vi "KH7008 Set All.vi"(8 "error in (no error)":errorcluster, 10 "Set All":T1={"Channel"=enum."Channel 2", "Gain"=enum."10x", "Bandwidth Filter"=enum."ON", "Shunt Resistor"=enum."50 Ohms", "Coupling"=enum."DC", "Input Config"=enum."Differential"}, 11 "VISA Refnum in":refnum<visa-resource-name>="COM1") -> (0 "error out":errorcluster)   [LabVIEW 2016, in "KH7008.lvclass"]
uses:
  KH7008.lvclass
  typedefs/SetAll-Cluster.ctl
  typedefs/Channel-Enum.ctl
  typedefs/Gain-Enum.ctl
  typedefs/Filter-Enum.ctl
  typedefs/Shunt-Enum.ctl
  typedefs/Coupling-Enum.ctl
  typedefs/Input Configuration-Enum.ctl
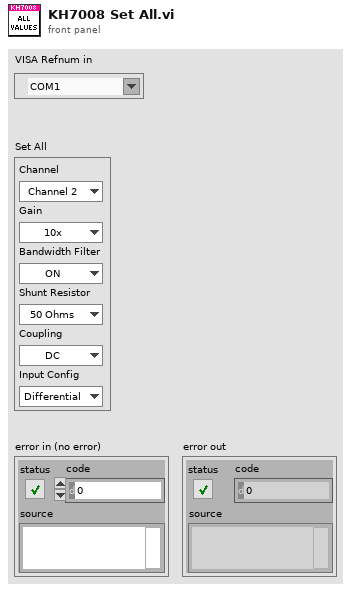
[diagram p1: front panel]
types:
  T1 = typedef "KH7008.lvclass/SetAll-Cluster.ctl" = cluster{"Channel":T2, "Gain":T3, "Bandwidth Filter":T4, "Shunt Resistor":T5, "Coupling":T6, "Input Config":T7}
  T2 = typedef "KH7008.lvclass/Channel-Enum.ctl" = enum16{"Channel 1", "Channel 2", "Channel 3", "Channel 4", "Channel 5", "Channel 6", "Channel 7", "Channel 8"}
  T3 = typedef "KH7008.lvclass/Gain-Enum.ctl" = enum16{"1x", "10x", "100x", "1000x"}
  T4 = typedef "KH7008.lvclass/Filter-Enum.ctl" = enum16{"OFF", "ON"}
  T5 = typedef "KH7008.lvclass/Shunt-Enum.ctl" = enum16{"Open", "50 Ohms", "500 Ohms", "5k Ohms", "50k Ohms"}
  T6 = typedef "KH7008.lvclass/Coupling-Enum.ctl" = enum16{"AC", "DC"}
  T7 = typedef "KH7008.lvclass/Input Configuration-Enum.ctl" = enum16{"Ground", "SE+ (-gnd)", "SE- (+gnd)", "Differential"}
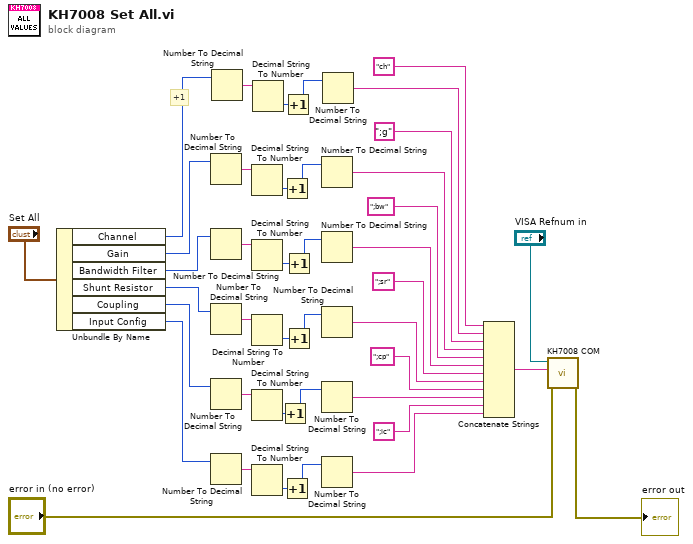
[diagram p0: block diagram]
diagram:
  # "+1"
  n1 = Unbundle By Name("Set All") -> ("Channel"=w6:T2, "Gain"=w33:T3, "Bandwidth Filter"=w32:T4, "Shunt Resistor"=w30:T5, "Coupling"=w31:T6, "Input Config"=w34:T7)
  n2 = Number To Decimal String(number=w33) -> (decimal integer string=w29:string)  [unwired: 1 in]
  n3 = Number To Decimal String(number=w32) -> (decimal integer string=w28:string)  [unwired: 1 in]
  n4 = Number To Decimal String(number=w30) -> (decimal integer string=w27:string)  [unwired: 1 in]
  n5 = Number To Decimal String(number=w31) -> (decimal integer string=w26:string)  [unwired: 1 in]
  n6 = Number To Decimal String(number=w34) -> (decimal integer string=w25:string)  [unwired: 1 in]
  n7 = Number To Decimal String(number=w6) -> (decimal integer string=w7:string)  [unwired: 1 in]
  n8 = Decimal String To Number(string=w29) -> (number=w24:i32)  [unwired: 2 in, 1 out]
  n9 = Decimal String To Number(string=w28) -> (number=w23:i32)  [unwired: 2 in, 1 out]
  n10 = Decimal String To Number(string=w27) -> (number=w20:i32)  [unwired: 2 in, 1 out]
  n11 = Decimal String To Number(string=w26) -> (number=w21:i32)  [unwired: 2 in, 1 out]
  n12 = Decimal String To Number(string=w25) -> (number=w22:i32)  [unwired: 2 in, 1 out]
  n13 = Decimal String To Number(string=w7) -> (number=w8:i32)  [unwired: 2 in, 1 out]
  n14 = Increment(x=w21) -> (x+1=w18:i32)
  n15 = Increment(x=w24) -> (x+1=w15:i32)
  n16 = Increment(x=w22) -> (x+1=w19:i32)
  n17 = Increment(x=w8) -> (x+1=w9:i32)
  n18 = Increment(x=w23) -> (x+1=w16:i32)
  n19 = Increment(x=w20) -> (x+1=w17:i32)
  n20 = Number To Decimal String(number=w15) -> (decimal integer string=w14:string)  [unwired: 1 in]
  n21 = Number To Decimal String(number=w16) -> (decimal integer string=w13:string)  [unwired: 1 in]
  n22 = Number To Decimal String(number=w17) -> (decimal integer string=w12:string)  [unwired: 1 in]
  n23 = Number To Decimal String(number=w18) -> (decimal integer string=w11:string)  [unwired: 1 in]
  n24 = Number To Decimal String(number=w19) -> (decimal integer string=w10:string)  [unwired: 1 in]
  n25 = Number To Decimal String(number=w9) -> (decimal integer string=w5:string)  [unwired: 1 in]
  n26 = Concatenate Strings("ch" ("string"), w5, ";g" ("string"), w14, ";bw" ("string"), w13, ";sr" ("string"), w12, ";cp" ("string"), w11, ";ic" ("string"), w10) -> (w41:string)
  n27 = call "KH7008 COM.vi"("error in (no error)"="error in (no error)", "Command"=w41, "VISA Refnum in"="VISA Refnum in") -> ("error out"=→"error out":errorcluster)  [unwired: 7 in, 1 out]
